vi "Display Timeout One Button Popup.vi"(6 "Theme":refnum<class "Theme.lvclass">, 7 "Button Text":string="OK", 8 "error in":errorcluster, 9 "Timeout (s)":dbl=1.0 min=1.0, 10 "Message":string, 11 "Graphic":T1="info") -> (0 "error out":errorcluster, 2 "Timeout":bool)   [LabVIEW 2021, in "Pop-Up.lvlib" / "Timeout One Button.lvclass"]
doc: "The one button popup will display information to the user and wait for the operator to click the button or until the timeout expires.\n\n<b>Note:</b> The function <b>Close Pop-Up.vi</b> can be used to close this dialog early.\n\nInputs: +\n-Graphic [typedef combobox] - Image (PNG) for Graphic for Popup +\n-Message [String] - String Variable to populate Display +\n-Theme [lvclass] - the theme for the style of the popup +\n-Timeout (s) [DBL] - the amount of seconds for the timeout +\n-Button Text [String] - the boolean text of the button\n\n<b>Code Developed By:</b> +\nDaniel Coons +\nhttps://github.com/danielcoons/tsc-pop-up"
uses:
  Timeout One Button.lvclass
  Graphics.ctl
  Theme/Theme.lvclass
  C:/Development/Open Source/tsc-pop-up/Popup/Popup.lvclass
  Timeout One Button.lvclass/Timeout One Button.ctl
  Popup/Popup.lvclass/Popup.ctl
  Popup/Popup.lvclass
  Pop-Up.lvlib
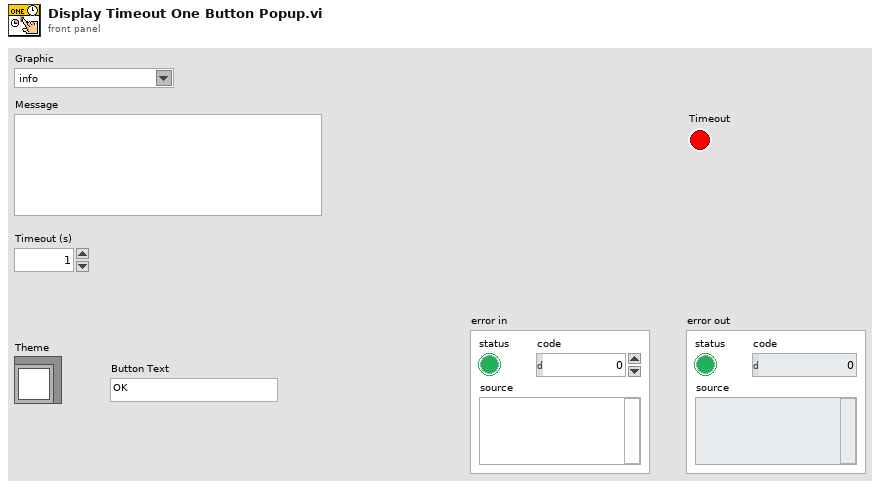
[diagram p1: front panel]
types:
  T1 = typedef "Pop-Up.lvlib/Graphics.ctl" = string
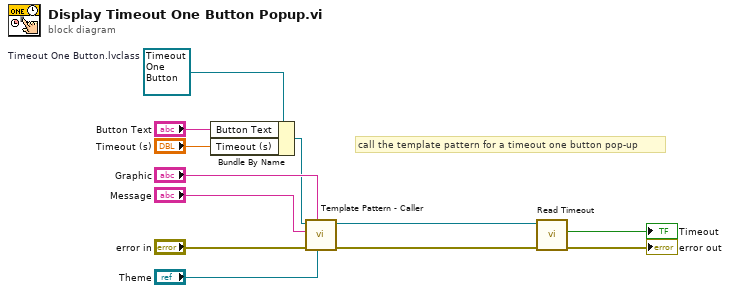
[diagram p0: block diagram]
diagram:
  w7 = refnum<class "Timeout One Button.lvclass"> refnum  # Timeout One Button.lvclass
  # "call the template pattern for a timeout one button pop-up"
  n1 = Bundle By Name(cluster=w7, "Button Text"="Button Text", "Timeout (s)"="Timeout (s)") -> (w8:refnum<class "Timeout One Button.lvclass">)
  n2 = call-dynamic "Template Pattern - Caller.vi"("Theme"="Theme", "standard"="Graphic", "error in (no error)"="error in", "Message"="Message", "Pop-Up in"=w8) -> ("error out"=w10:errorcluster, "Pop-Up out"=w2:refnum<class "Timeout One Button.lvclass">)  [unwired: 5 in]
  n3 = call "Read Timeout.vi"("error in"=w10, "Popup in"=w2) -> ("error out"=→"error out":errorcluster, "Timeout?"=→"Timeout":bool)  [unwired: 7 in, 1 out]
